vi "Data Type to Assert.vi"(8 "error in (no error)":errorcluster, 11 "Data Type":refnum<class "Data Type.lvclass">) -> (0 "error out":errorcluster, 3 "Assert":refnum<class "Assert.lvclass">)   [LabVIEW 2019, in "Assertion.lvclass"]
uses:
  <vilib>/gpm_packages/@cs/data-type-serializer/source/Assertion/Assertion.lvclass
  <vilib>/gpm_packages/@cs/data-type-serializer/source/Data Type/Data Type.lvclass
  <vilib>/gpm_packages/@cs/run-time-assertions/Source/Assert/Assert.lvclass
  <vilib>/gpm_packages/@cs/data-type-serializer/source/Assertion/Assertion.lvclass/Assertion.ctl
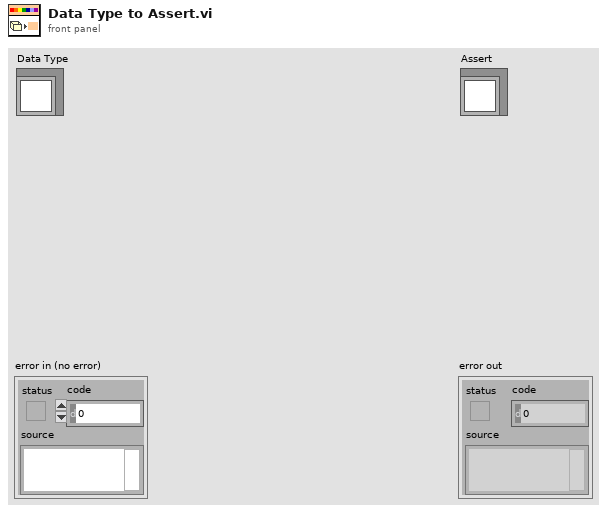
[diagram p1: front panel]
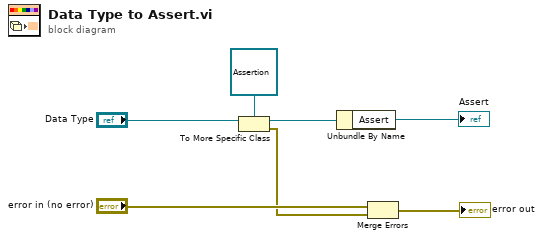
[diagram p0: block diagram]
diagram:
  n1 = To More Specific Class(target class=refnum<class "Assertion.lvclass"> refnum ("Boolean out"), reference="Data Type") -> (specific class reference=w4:refnum<class "Assertion.lvclass">, error out=w2:errorcluster)  [unwired: 1 in]
  n2 = Unbundle By Name(w4) -> ("Assert"=→"Assert":refnum<class "Assert.lvclass">)
  n3 = Merge Errors("error in (no error)", w2) -> (→"error out":errorcluster)
